vi "Initialize configuration property (interaction).vi"(6 "vsChIndex":i32, 9 "parameter name":string, 10 "datatype":string, 11 "interaction class name":string) -> (3 "attribute configuration":T1)   [LabVIEW 2019, in "HLA Custom Device System Explorer.lvlib"]
uses:
  HLA Custom Device System Explorer.lvlib
  Shared/interaction_parameter_configuration.ctl
  Shared/HLA Custom Device Shared.lvlib
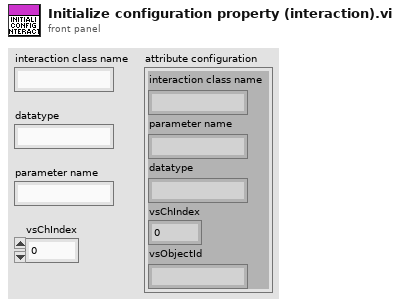
[diagram p1: front panel]
types:
  T1 = typedef "HLA Custom Device Shared.lvlib/interaction_parameter_configuration.ctl" = cluster{"interaction class name":string, "parameter name":string, "datatype":string, "vsChIndex":i32, "vsObjectId":string}
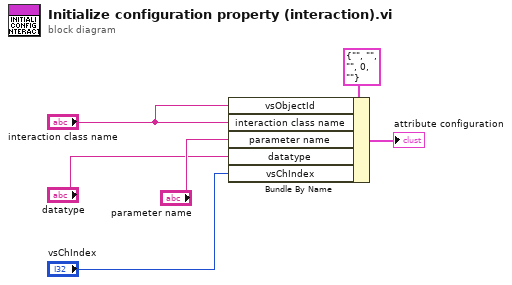
[diagram p0: block diagram]
diagram:
  n1 = Bundle By Name(cluster=T1 {"interaction class name"="", "parameter name"="", "datatype"="", "vsChIndex"=0, "vsObjectId"=""}, "vsObjectId"="interaction class name", "interaction class name"="interaction class name", "parameter name"="parameter name", "datatype"="datatype", "vsChIndex"="vsChIndex") -> (→"attribute configuration":T1)
